vi "Actions FG.vi"(10 "Action Name":string) -> (0 "error out":errorcluster, 2 "Action":refnum<class "CLIAction.lvclass">)   [LabVIEW 2020, in "GPackTools.lvlib"]
uses:
  GPackTools.lvlib
  CLIAction/CLIAction.lvclass
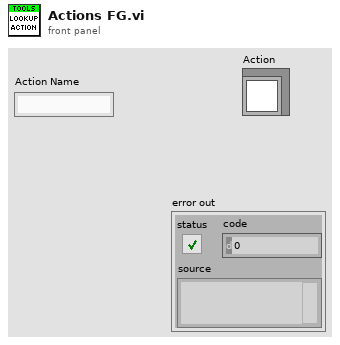
[diagram p1: front panel]
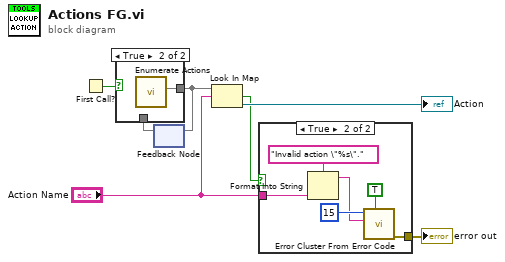
[diagram p0: block diagram]
diagram:
  n1 = First Call?() -> (First Call?: T/F=w7:bool)
  n2 = feedback #1() -> (w6:map{string, refnum<class "CLIAction.lvclass">})  [unwired: 1 in]
  n3 = case shown="True" w7 {
    tunnel: [w8 w9] -> w5
    tunnel: w6 -> [w8 _]
    frame False {
    }
    frame True {
      n4 = call "Enumerate Actions.vi"() -> ("Actions"=w9:map{string, refnum<class "CLIAction.lvclass">})  [unwired: 11 in]
    }
  }
  n5 = feedback-in #1(w5) -> ()
  n6 = Look In Map(map=w5, key="Action Name") -> (key not found?=w3:bool, value=→"Action":refnum<class "CLIAction.lvclass">)  [unwired: 1 in]
  n7 = case shown="True" w3 {
    tunnel: "Action Name" -> [_ w15]
    tunnel: [_ w10] -> w1
    frame False {
    }
    frame True {
      n8 = Format Into String(format string="Invalid action \"%s\".", w15) -> (resulting string=w11:string)  [unwired: 2 in, 1 out]
      n9 = call <vilib>:"Error Cluster From Error Code.vi"("show call chain? (False)"=TRUE, "error message (\"\")"=w11, "error code (0)"=15) -> ("error out"=w10:errorcluster)  [unwired: 6 in]
    }
  }
  "error out" <- w1
